vi "GetMetricIds.vi"(8 "metrics":T1[](array[typedef]), 9 "device type config":T13[](array[typedef]), 10 "AssetNodes":T3[](array[typedef]), 11 "channels":T14[](array[typedef])) -> (3 "metric ids":string[](array[string]))   [LabVIEW 2017, in "GlobalConfiguration.lvlib"]
uses:
  <vilib>/addons/InsightCM/Utilities/GlobalConfiguration/GlobalConfiguration.lvlib
  <vilib>/addons/InsightCM/MessageBus/Base/controls/R2_Channel.ctl
  <vilib>/addons/InsightCM/MessageBus/Base/controls/KeyValuePair.ctl
  <vilib>/addons/InsightCM/MessageBus/Base/controls/Metric.ctl
  <vilib>/addons/InsightCM/MessageBus/Base/controls/SectionKeyValues.ctl
  <vilib>/addons/InsightCM/MessageBus/Base/controls/AssetNode.ctl
  <vilib>/addons/InsightCM/MessageBus/Base/controls/AssetState.ctl
  <vilib>/addons/InsightCM/MessageBus/Base/controls/OperatingState.ctl
  <vilib>/addons/InsightCM/MessageBus/Base/controls/Trigger.ctl
  <vilib>/addons/InsightCM/MessageBus/Base/controls/Condition.ctl
  <vilib>/addons/InsightCM/MessageBus/Base/controls/TrendAlarmRule.ctl
  <vilib>/addons/InsightCM/MessageBus/Base/controls/TrendAlarmLevel.ctl
  <vilib>/addons/InsightCM/MessageBus/Base/controls/AlarmAction.ctl
  <vilib>/addons/InsightCM/MessageBus/Base/controls/AssetNodeReference.ctl
  <vilib>/addons/InsightCM/MessageBus/Base/controls/MetricDefinitionInstance.ctl
  <vilib>/addons/InsightCM/Utilities/PropertyHelpers/PropertyHelpers.lvlib
  <vilib>/addons/InsightCM/Utilities/DeviceModelHelpers/DeviceModelHelpers.lvlib
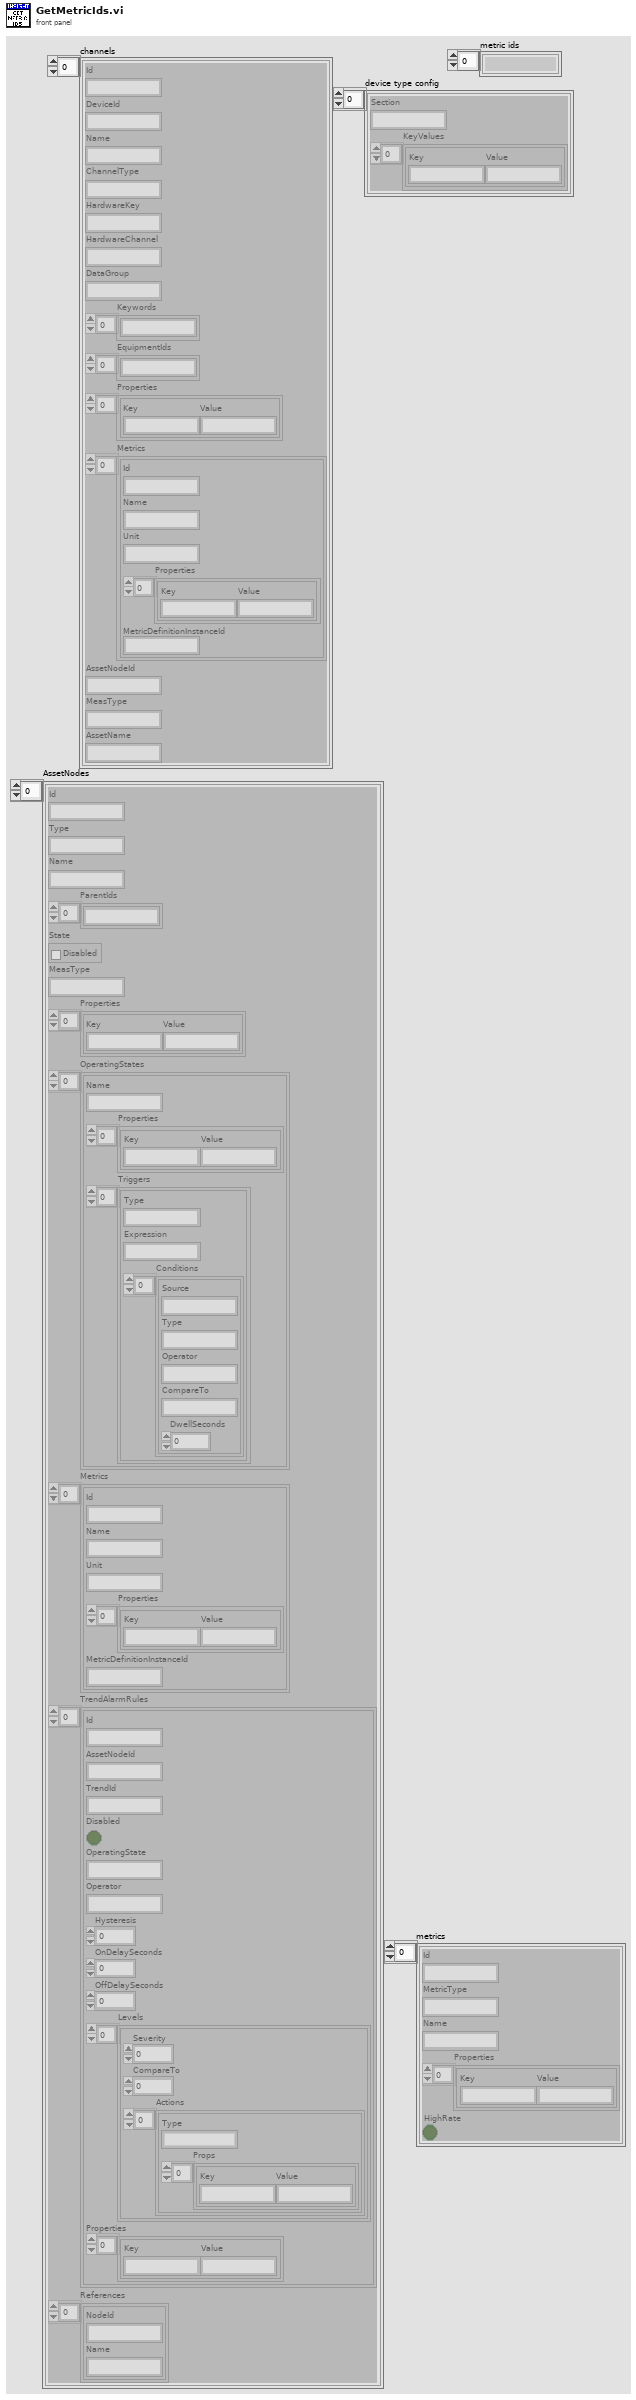
[diagram p1: front panel]
types:
  T1 = typedef "MetricDefinitionInstance.ctl" = cluster{"Id":string, "MetricType":string, "Name":string, "Properties":T2[], "HighRate":bool}
  T2 = typedef "KeyValuePair.ctl" = cluster{"Key":string, "Value":string}
  T3 = typedef "AssetNode.ctl" = cluster{"Id":string, "Type":string, "Name":string, "ParentIds":string[], "State":T4, "MeasType":string, "Properties":T2[], "OperatingStates":T5[], "Metrics":T8[], "TrendAlarmRules":T9[], "References":T12[]}
  T4 = typedef "AssetState.ctl" = cluster{"Disabled":bool}
  T5 = typedef "OperatingState.ctl" = cluster{"Name":string, "Properties":T2[], "Triggers":T6[]}
  T6 = typedef "Trigger.ctl" = cluster{"Type":string, "Expression":string, "Conditions":T7[]}
  T7 = typedef "Condition.ctl" = cluster{"Source":string, "Type":string, "Operator":string, "CompareTo":string, "DwellSeconds":dbl}
  T8 = typedef "Metric.ctl" = cluster{"Id":string, "Name":string, "Unit":string, "Properties":T2[], "MetricDefinitionInstanceId":string}
  T9 = typedef "TrendAlarmRule.ctl" = cluster{"Id":string, "AssetNodeId":string, "TrendId":string, "Disabled":bool, "OperatingState":string, "Operator":string, "Hysteresis":dbl, "OnDelaySeconds":dbl, "OffDelaySeconds":dbl, "Levels":T10[], "Properties":T2[]}
  T10 = typedef "TrendAlarmLevel.ctl" = cluster{"Severity":i32, "CompareTo":dbl, "Actions":T11[]}
  T11 = typedef "AlarmAction.ctl" = cluster{"Type":string, "Props":T2[]}
  T12 = typedef "AssetNodeReference.ctl" = cluster{"NodeId":string, "Name":string}
  T13 = typedef "SectionKeyValues.ctl" = cluster{"Section":string, "KeyValues":T2[]}
  T14 = typedef "R2_Channel.ctl" = cluster{"Id":string, "DeviceId":string, "Name":string, "ChannelType":string, "HardwareKey":string, "HardwareChannel":string, "DataGroup":string, "Keywords":string[], "EquipmentIds":string[], "Properties":T2[], "Metrics":T8[], "AssetNodeId":string, "MeasType":string, "AssetName":string}
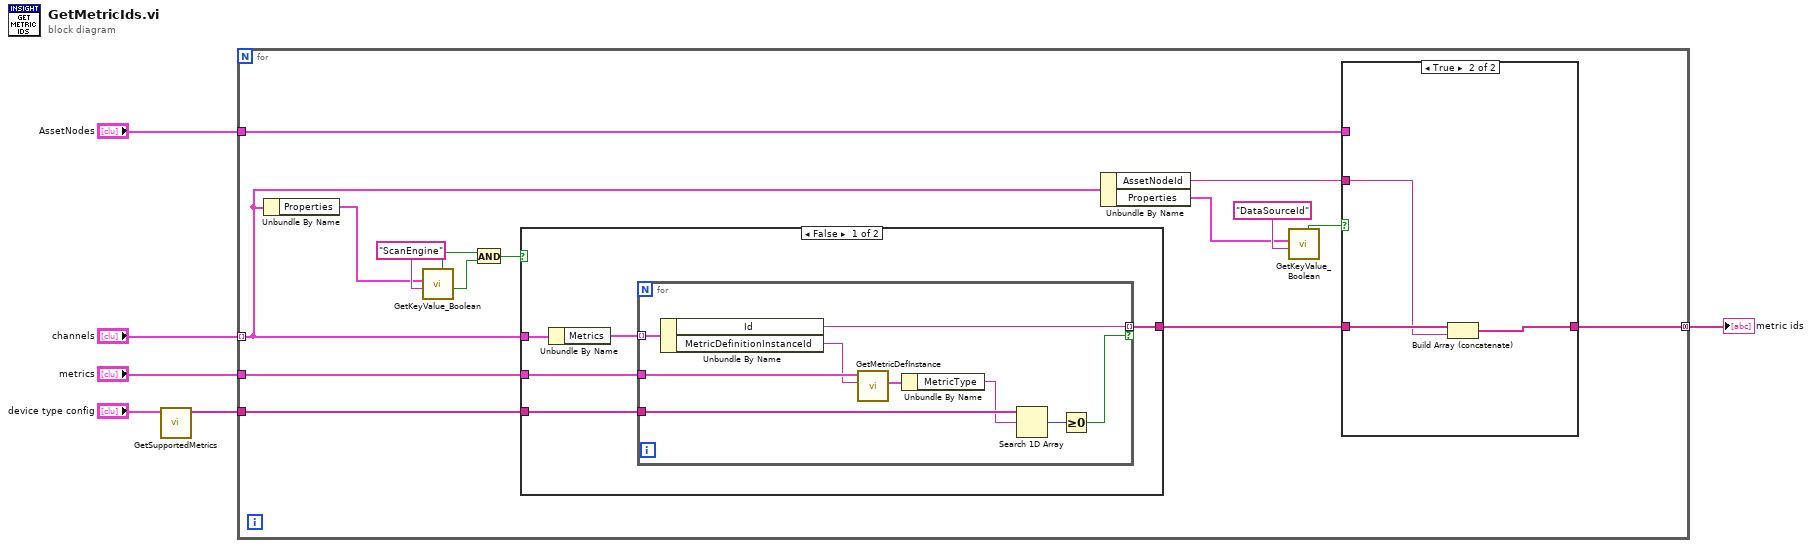
[diagram p0: block diagram]
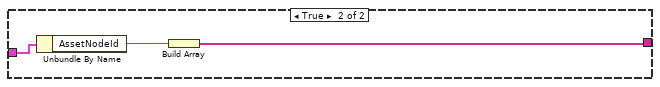
[diagram p3: hidden frame]
diagram:
  n1 = call <vilib>:"GetSupportedMetrics.vi"("key values"="device type config") -> ("supported metrics"=w4:string[])  [unwired: 10 in]
  n2 = for {
    tunnel: "channels" -> [w12] mode=indexing
    tunnel: w4 -> [w17]
    tunnel: [w7] -> w3 mode=concatenating
    tunnel: "AssetNodes" -> [w10]
    tunnel: "metrics" -> [w9]
    n3 = Unbundle By Name(w12) -> ("Properties"=w16:T2[])
    n4 = call <vilib>:"GetKeyValue_Boolean.vi"("key"="ScanEngine", "key value pairs"=w16) -> ("value"=w19:bool, "found"=w20:bool)  [unwired: 7 in, 1 out]
    n5 = And(x=w20, y=w19) -> (x .and. y?=w18:bool)
    n6 = case shown="False" w18 {
      tunnel: w12 -> [w30 w42]
      tunnel: [w28 w40] -> w8
      tunnel: w17 -> [w27 _]
      tunnel: w9 -> [w26 _]
      frame False {
        n7 = Unbundle By Name(w30) -> ("Metrics"=w29:T8[])
        n8 = for {
          tunnel: w29 -> [w39] mode=indexing
          tunnel: [w38] -> w28 mode=indexing if=w35
          tunnel: w27 -> [w37]
          tunnel: w26 -> [w34]
          n9 = Unbundle By Name(w39) -> ("Id"=w38:string, "MetricDefinitionInstanceId"=w32:string)
          n10 = call <vilib>:"GetMetricDefInstance.vi"("metric definition instance id"=w32, "metric definition instances"=w34) -> ("metric definition instance"=w33:T1)  [unwired: 7 in, 2 out]
          n11 = Unbundle By Name(w33) -> ("MetricType"=w31:string)
          n12 = Search 1D Array(1D array=w37, element=w31) -> (index of element=w36:i32)  [unwired: 1 in]
          n13 = Greater Or Equal To 0?(x=w36) -> (x >= 0?=w35:bool)
        }
      }
      frame True {
        n14 = Unbundle By Name(w42) -> ("AssetNodeId"=w41:string)
        n15 = Build Array(w41) -> (w40:string[])
      }
    }
    n16 = Unbundle By Name(w12) -> ("AssetNodeId"=w11:string, "Properties"=w13:T2[])
    n17 = call <vilib>:"GetKeyValue_Boolean.vi"("key"="DataSourceId", "key value pairs"=w13) -> ("found"=w14:bool)  [unwired: 7 in, 2 out]
    n18 = case shown="True" w14 {
      tunnel: w11 -> [_ w24]
      tunnel: w10 -> [_ _]
      tunnel: w8 -> [w22 w25]
      tunnel: [w22 w23] -> w7
      frame False {
      }
      frame True {
        n19 = Build Array (concatenate)(w25, w24) -> (w23:string[])
      }
    }
  }
  "metric ids" <- w3
